vi "0716206_calculator.vi"() -> ()   [LabVIEW 2021]
uses:
  <vilib>/gmath/NI_Gmath.lvlib
panel:
  out "Power":bool
  out "Storage2 ans":dbl format="%#_13g"
  out "Storage1 ans":dbl format="%#_13g"
  out "B":bool=TRUE
  out "Storage2":string
  out "Storage1":string
  out "Error":string
  out "Ans":dbl format="%#_13g"
  out "System Time":string
  out "Execution Time (s)":dbl caption="Elapsed Time (s)"
  out "String":string
  in  "Cluster":T1
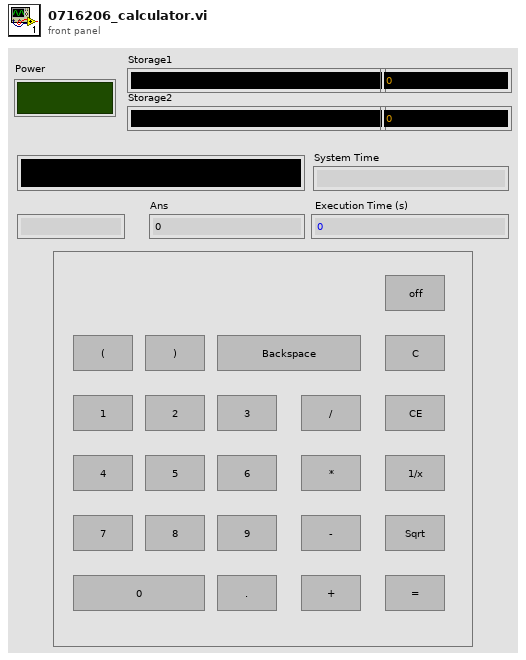
[diagram p1: front panel]
types:
  T1 = cluster{bool, bool, bool, bool, bool, bool, bool, bool, bool, bool, bool, bool, bool, bool, bool, bool, bool, bool, bool, bool, bool, bool, bool, bool}
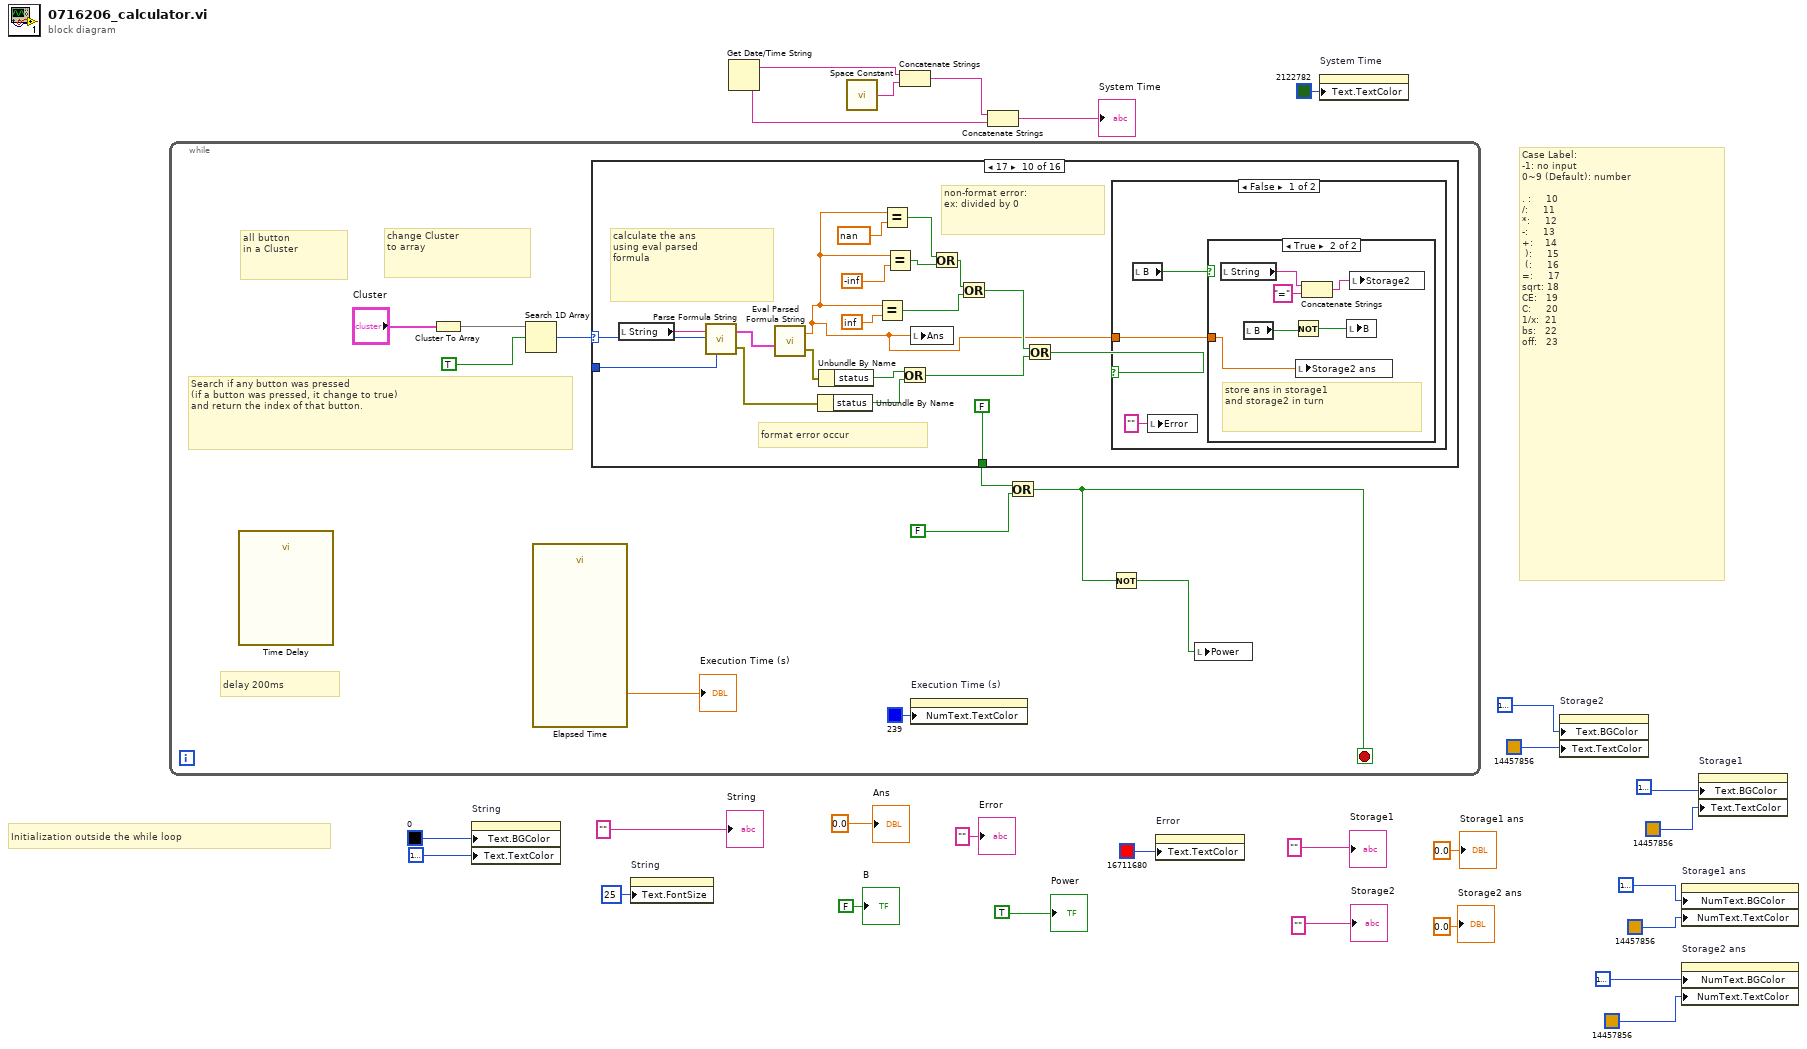
[diagram p0: block diagram]
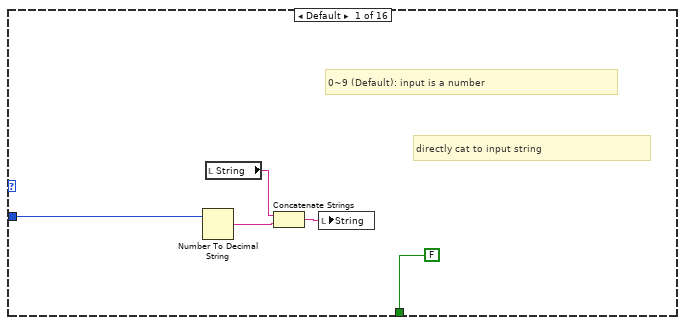
[diagram p2: hidden frame]
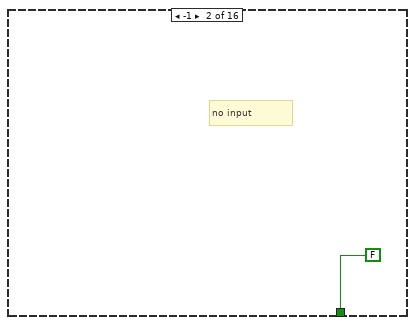
[diagram p3: hidden frame]
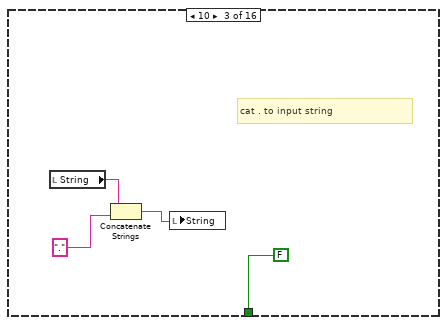
[diagram p4: hidden frame]
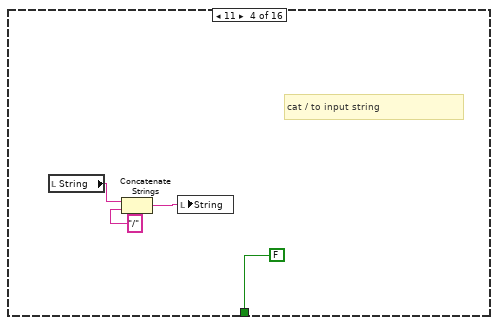
[diagram p5: hidden frame]
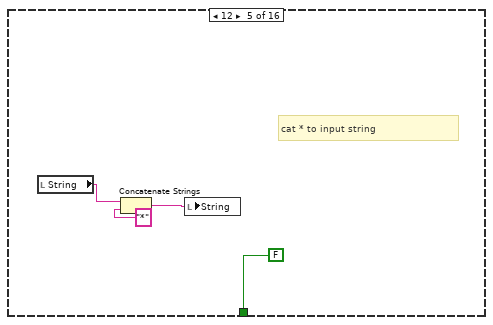
[diagram p6: hidden frame]
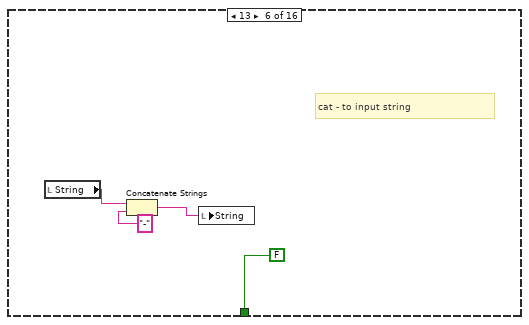
[diagram p7: hidden frame]
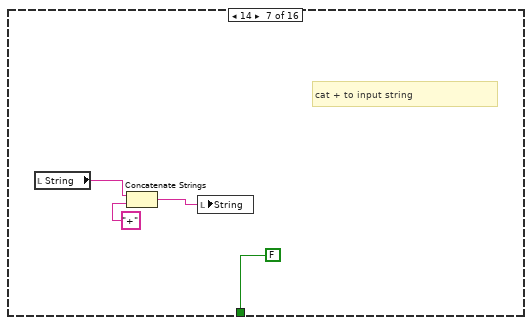
[diagram p8: hidden frame]
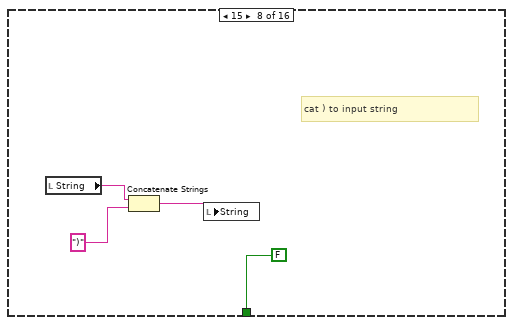
[diagram p9: hidden frame]
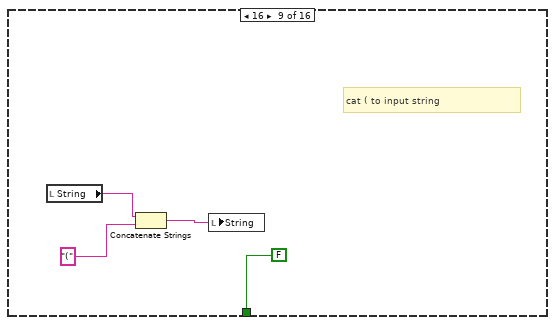
[diagram p10: hidden frame]
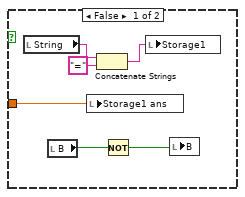
[diagram p11: hidden frame]
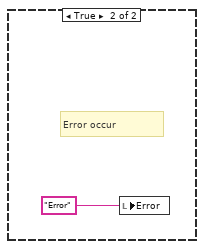
[diagram p12: hidden frame]
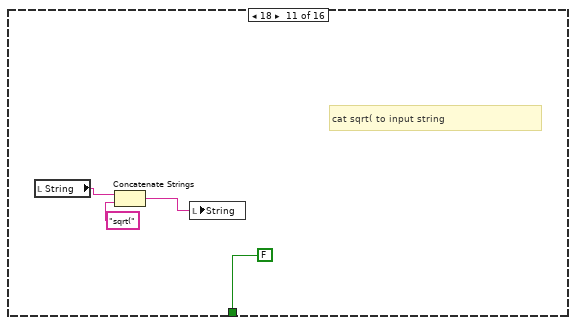
[diagram p13: hidden frame]
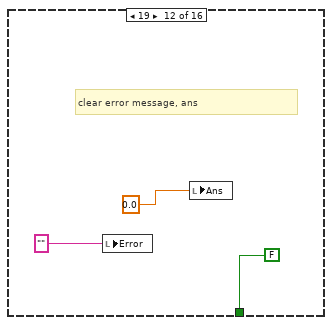
[diagram p14: hidden frame]
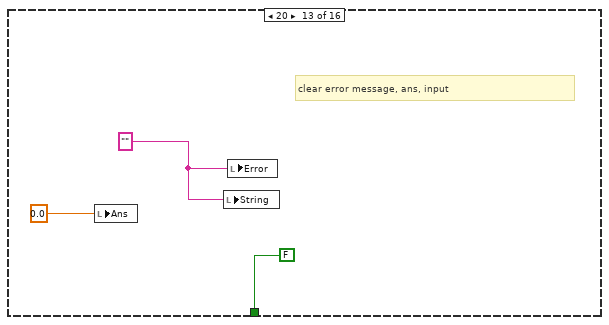
[diagram p15: hidden frame]
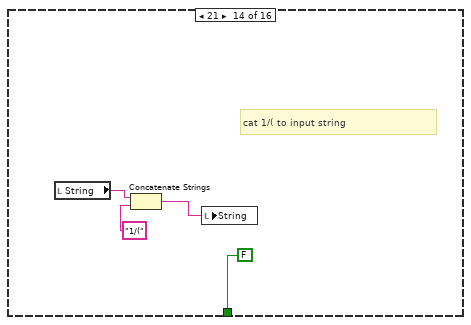
[diagram p16: hidden frame]
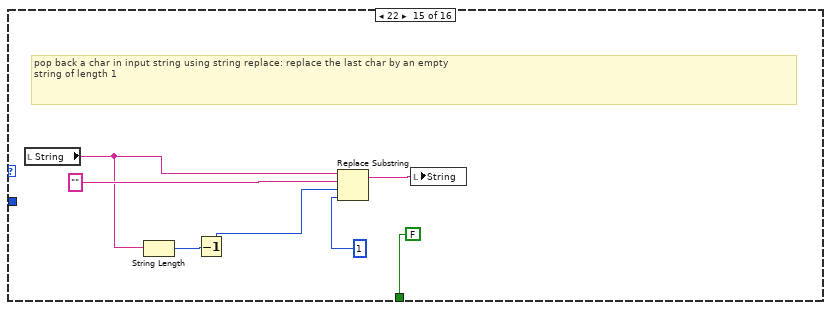
[diagram p17: hidden frame]
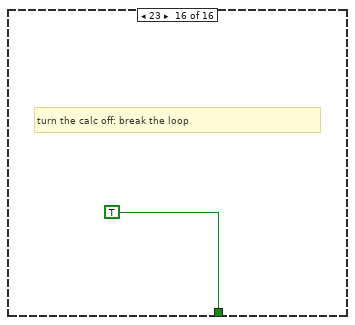
[diagram p18: hidden frame]
diagram:
  # "Initialization outside the while loop"
  # "Case Label:\n-1: no input\n0~9 (Default): number\n\n. :     10\n/:     11\n*:     12\n-:     13\n+:    14\n ):     15\n (:     16\n=:     17\nsqrt: 18\nCE:   19\nC:     20\n1/x:  21\nbs:   22\noff:   23"
  n1 = while {
    stop <- w28 stop-if-true
    # "Search if any button was pressed\n(if a button was pressed, it change to true)\nand return the index of that button."
    # "change Cluster \nto array"
    # "all button \nin a Cluster"
    # "delay 200ms"
    n2 = call "Time Delay"() -> ()  [unwired: 11 in, 1 out]
    n3 = Cluster To Array(cluster="Cluster") -> (array=w36:bool[])
    n4 = Search 1D Array(1D array=w36, element=TRUE) -> (index of element=w34:i32)  [unwired: 1 in]
    n5 = call "Elapsed Time"() -> ("Elapsed Time (s)"=→"Execution Time (s)":dbl)  [unwired: 12 in, 7 out]
    n6 = case shown="17" w34 {
      tunnel: w34 -> [w39 _ _ _ _ _ _ _ _ _ _ _ _ _ _ _]
      tunnel: [FALSE FALSE FALSE FALSE FALSE FALSE FALSE FALSE FALSE FALSE FALSE FALSE FALSE FALSE FALSE TRUE] -> w33
      frame Default {
        # "directly cat to input string"
        # "0~9 (Default): input is a number"
        n7 = Number To Decimal String(number=w39) -> (decimal integer string=w40:string)  [unwired: 1 in]
        n8 = local read "String"() -> (w41:string)
        n9 = Concatenate Strings(w41, w40) -> (w42:string)
        n10 = local write "String"(w42) -> ()
      }
      frame -1 {
        # "no input"
      }
      frame 10 {
        # "cat . to input string"
        n11 = local read "String"() -> (w47:string)
        n12 = Concatenate Strings(w47, "." ("string")) -> (w46:string)
        n13 = local write "String"(w46) -> ()
      }
      frame 11 {
        # "cat / to input string"
        n14 = local read "String"() -> (w51:string)
        n15 = Concatenate Strings(w51, "/" ("string")) -> (w49:string)
        n16 = local write "String"(w49) -> ()
      }
      frame 12 {
        # "cat * to input string"
        n17 = local read "String"() -> (w55:string)
        n18 = Concatenate Strings(w55, "*" ("string")) -> (w53:string)
        n19 = local write "String"(w53) -> ()
      }
      frame 13 {
        # "cat - to input string"
        n20 = local read "String"() -> (w59:string)
        n21 = Concatenate Strings(w59, "-" ("string")) -> (w57:string)
        n22 = local write "String"(w57) -> ()
      }
      frame 14 {
        # "cat + to input string"
        n23 = local read "String"() -> (w63:string)
        n24 = Concatenate Strings(w63, "+" ("string")) -> (w62:string)
        n25 = local write "String"(w62) -> ()
      }
      frame 15 {
        # "cat ) to input string"
        n26 = local read "String"() -> (w66:string)
        n27 = Concatenate Strings(w66, ")" ("string")) -> (w67:string)
        n28 = local write "String"(w67) -> ()
      }
      frame 16 {
        # "cat ( to input string"
        n29 = local read "String"() -> (w70:string)
        n30 = Concatenate Strings(w70, "(" ("string")) -> (w71:string)
        n31 = local write "String"(w71) -> ()
      }
      frame 17 {
        # "non-format error:\nex: divided by 0"
        # "format error occur"
        # "calculate the ans\nusing eval parsed\nformula"
        n32 = local read "String"() -> (w89:string)
        n33 = call <vilib>:"Parse Formula String.vi"("formula"=w89) -> ("error out"=w86:errorcluster, "Parsed Formula"=w88:cluster{"Table":i32[][], "Y Values":dbl[]})  [unwired: 1 in]
        n34 = call <vilib>:"Eval Parsed Formula String.vi"("Parsed Formula"=w88) -> ("error out"=w85:errorcluster, "y value"=w72:dbl)  [unwired: 3 in]
        n35 = Unbundle By Name(w86) -> ("status"=w83:bool)
        n36 = Unbundle By Name(w85) -> ("status"=w84:bool)
        n37 = Equal?(x=w72, y=inf) -> (x = y?=w77:bool)
        n38 = Equal?(x=w72, y=nan) -> (x = y?=w73:bool)
        n39 = Equal?(x=w72, y=-inf) -> (x = y?=w79:bool)
        n40 = Or(x=w84, y=w83) -> (x .or. y?=w75:bool)
        n41 = local write "Ans"(w72) -> ()
        n42 = Or(x=w73, y=w79) -> (x .or. y?=w78:bool)
        n43 = Or(x=w78, y=w77) -> (x .or. y?=w76:bool)
        n44 = Or(x=w76, y=w75) -> (x .or. y?=w74:bool)
        n45 = case shown="False" w74 {
          tunnel: w72 -> [w90 _]
          frame False {
            n46 = local read "B"() -> (w91:bool)
            n47 = local write "Error"("" ("Error")) -> ()
            n48 = case shown="True" w91 {
              tunnel: w90 -> [w93 w99]
              frame False {
                n49 = local read "String"() -> (w96:string)
                n50 = local read "B"() -> (w98:bool)
                n51 = local write "Storage1 ans"(w93) -> ()
                n52 = Concatenate Strings(w96, "=" ("string")) -> (w94:string)
                n53 = Not(x=w98) -> (.not. x?=w97:bool)
                n54 = local write "Storage1"(w94) -> ()
                n55 = local write "B"(w97) -> ()
              }
              frame True {
                # "store ans in storage1 \nand storage2 in turn"
                n56 = local read "String"() -> (w102:string)
                n57 = local read "B"() -> (w104:bool)
                n58 = Not(x=w104) -> (.not. x?=w103:bool)
                n59 = local write "Storage2 ans"(w99) -> ()
                n60 = Concatenate Strings(w102, "=" ("string")) -> (w100:string)
                n61 = local write "B"(w103) -> ()
                n62 = local write "Storage2"(w100) -> ()
              }
            }
          }
          frame True {
            # "Error occur"
            n63 = local write "Error"("Error" ("Error")) -> ()
          }
        }
      }
      frame 18 {
        # "cat sqrt( to input string"
        n64 = local read "String"() -> (w108:string)
        n65 = Concatenate Strings(w108, "sqrt(" ("string")) -> (w109:string)
        n66 = local write "String"(w109) -> ()
      }
      frame 19 {
        # "clear error message, ans"
        n67 = local write "Error"("" ("Error")) -> ()
        n68 = local write "Ans"(0.0 ("Ans")) -> ()
      }
      frame 20 {
        w113 = "" ("String")
        # "clear error message, ans, input"
        n69 = local write "Ans"(0.0 ("Ans")) -> ()
        n70 = local write "String"(w113) -> ()
        n71 = local write "Error"(w113) -> ()
      }
      frame 21 {
        # "cat 1/( to input string"
        n72 = local read "String"() -> (w118:string)
        n73 = Concatenate Strings(w118, "1/(" ("string")) -> (w119:string)
        n74 = local write "String"(w119) -> ()
      }
      frame 22 {
        # "pop back a char in input string using string replace: replace the last char by an empty\nstring of length 1"
        n75 = local read "String"() -> (w121:string)
        n76 = String Length(string=w121) -> (length=w124:i32)
        n77 = Decrement(x=w124) -> (x-1=w125:i32)
        n78 = Replace Substring(2:1 ("length (len. of substring)"), 3:w125, 4:"" ("substring (\"\")"), 5:w121) -> (1:w126:string)  [unwired: 1 out]
        n79 = local write "String"(w126) -> ()
      }
      frame 23 {
        # "turn the calc off: break the loop"
      }
    }
    n80 = property on="Execution Time (s)" class="DigNum (strict)"("NumText.TextColor"=u32 239 ("Numeric Text.Text Colors:Text Color")) -> ()  [unwired: 2 in, 2 out]
    n81 = Or(x=w33, y=FALSE) -> (x .or. y?=w28:bool)
    n82 = Not(x=w28) -> (.not. x?=w29:bool)
    n83 = local write "Power"(w29) -> ()
  }
  n84 = property on="String" class="Str"("Text.BGColor"=u32 0 ("Text.Text Colors:BG Color"), "Text.TextColor"=u32 16777238 ("Text.Text Colors:Text Color")) -> ()  [unwired: 2 in, 2 out]
  n85 = property on="String" class="Str"("Text.FontSize"=u32 25 ("Text.Font:Size")) -> ()  [unwired: 2 in, 2 out]
  n86 = Get Date/Time String() -> (date string=w25:string, time string=w23:string)  [unwired: 3 in]
  n87 = call <vilib>:"Space Constant.vi"() -> ("String"=w26:string)
  n88 = Concatenate Strings(w25, w26) -> (w24:string)
  n89 = Concatenate Strings(w24, w23) -> (→"System Time":string)
  n90 = property on="Error" class="Str"("Text.TextColor"=u32 16711680 ("Text.Text Colors:Text Color")) -> ()  [unwired: 2 in, 2 out]
  n91 = property on="System Time" class="Str"("Text.TextColor"=u32 2122782 ("Text.Text Colors:Text Color")) -> ()  [unwired: 2 in, 2 out]
  n92 = property on="Storage2" class="Str"("Text.BGColor"=u32 16777222 ("Text.Text Colors:BG Color"), "Text.TextColor"=u32 14457856 ("Text.Text Colors:Text Color")) -> ()  [unwired: 2 in, 2 out]
  n93 = property on="Storage1 ans" class="DigNum (strict)"("NumText.BGColor"=u32 16777222 ("Text.Text Colors:BG Color"), "NumText.TextColor"=u32 14457856 ("Text.Text Colors:Text Color")) -> ()  [unwired: 2 in, 2 out]
  n94 = property on="Storage2 ans" class="DigNum (strict)"("NumText.BGColor"=u32 16777222 ("Text.Text Colors:BG Color"), "NumText.TextColor"=u32 14457856 ("Text.Text Colors:Text Color")) -> ()  [unwired: 2 in, 2 out]
  n95 = property on="Storage1" class="Str"("Text.BGColor"=u32 16777222 ("Text.Text Colors:BG Color"), "Text.TextColor"=u32 14457856 ("Text.Text Colors:Text Color")) -> ()  [unwired: 2 in, 2 out]
  "String" <- ""
  "Ans" <- 0.0 ("Ans")
  "Error" <- "" ("Error")
  "Storage1" <- ""
  "Storage2" <- ""
  "B" <- FALSE ("Boolean")
  "Storage1 ans" <- 0.0 ("Storage1 ans")
  "Storage2 ans" <- 0.0 ("Storage2 ans")
  "Power" <- TRUE ("Power")
